vi "Sample Rate To Loop Time.vi"   [LabVIEW 2017, in "NI_FpgaMspHost.lvlib"]
doc: "Converts the desired sample rate to the appropriate count for the Loop Timer Express VI and computes the achievable sample rate for use with other Scaling VIs."
uses:
  <vilib>/rvi/Analysis/host/Public/NI_FpgaMspHost.lvlib
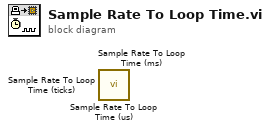
[diagram p0: block diagram]
diagram:
  n1 = call <vilib>:"Sample Rate To Loop Time (us).vi"() -> ()  [unwired: 13 in, 3 out]
  n2 = call <vilib>:"Sample Rate To Loop Time (ms).vi"() -> ()  [unwired: 13 in, 3 out]
  n3 = call <vilib>:"Sample Rate To Loop Time (ticks).vi"() -> ()  [unwired: 13 in, 3 out]
